vi "Check_Vol_Mounted.vi"(0 "Filename":path) -> (1 "Filename Out":path, 2 "exists?":bool)   [LabVIEW 2010]
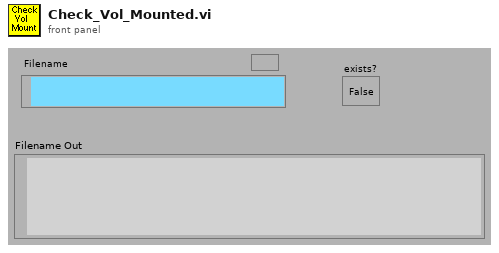
[diagram p1: front panel]
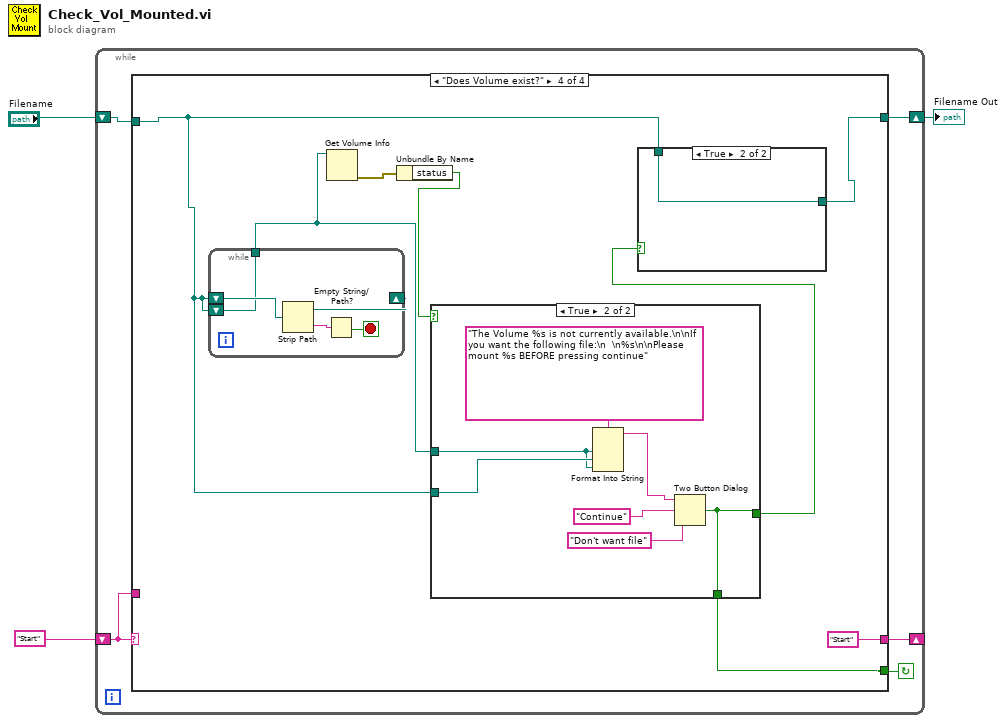
[diagram p0: block diagram]
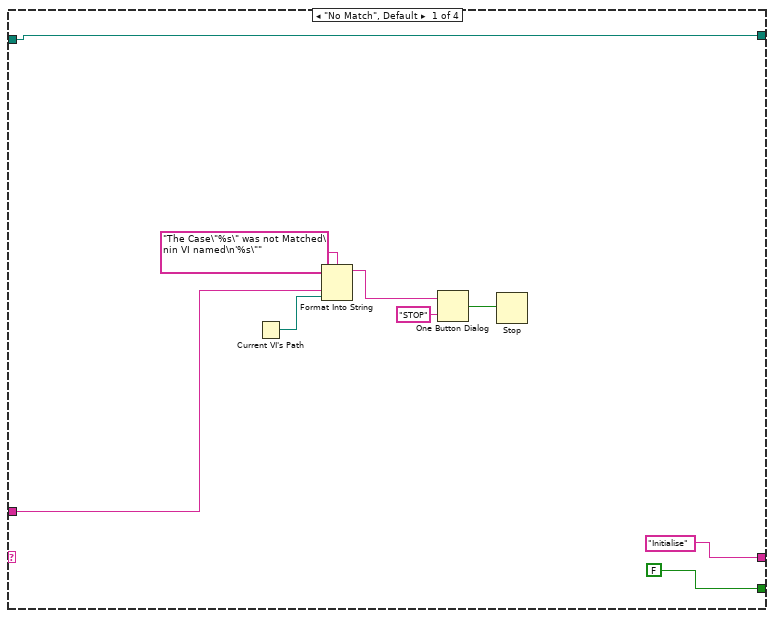
[diagram p2: hidden frame]
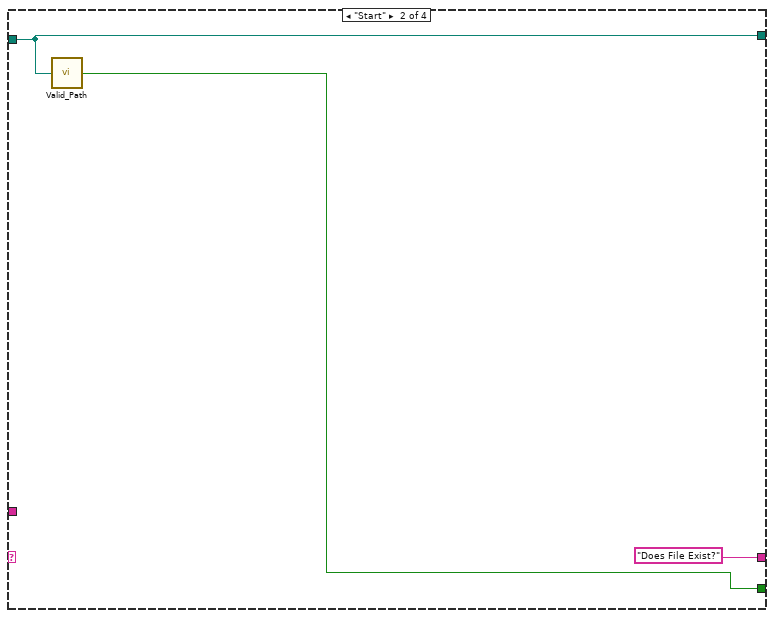
[diagram p3: hidden frame]
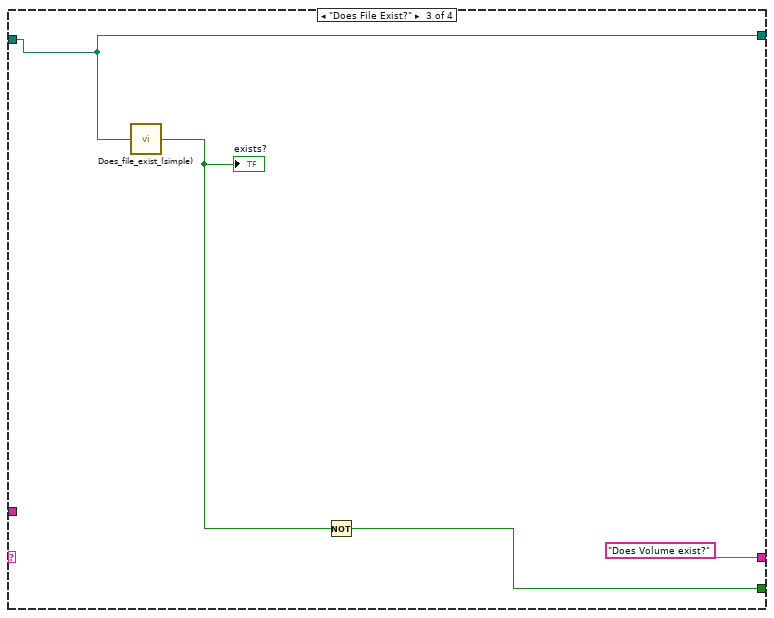
[diagram p4: hidden frame]
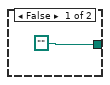
[diagram p5: hidden frame]
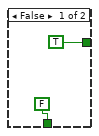
[diagram p6: hidden frame]
diagram:
  n1 = while {
    shift-left: "Start" -> [w6]
    shift-right: [w7] -> _
    shift-right: [w4] -> w1
    shift-left: "Filename" -> [w5]
    stop <- w8 continue-if-true
    n2 = case shown="\"Does Volume exist?\"" w6 {
      tunnel: [FALSE w19 w22 w26] -> w8
      tunnel: ["Initialise" "Does File Exist?" "Does Volume exist?" "Start"] -> w7
      tunnel: w6 -> [w12 _ _ _]
      tunnel: w5 -> [w9 w18 w21 w25]
      tunnel: [w9 w18 w21 w28] -> w4
      frame "No Match", Default {
        n3 = Current VI's Path() -> (path=w11:path)
        n4 = Format Into String(format string="The Case\"%s\" was not Matched\nin VI named\n'%s\"" ("Format String"), w12, w11) -> (resulting string=w15:string)  [unwired: 2 in, 1 out]
        n5 = One Button Dialog(message=w15, button name ("OK")="STOP") -> (true=w13:bool)
        n6 = Stop(stop? (T)=w13) -> ()
      }
      frame "Start" {
        n7 = call "Valid_Path.vi"("Filename"=w18) -> ("Valid Path?"=w19:bool)
      }
      frame "Does File Exist?" {
        n8 = call "Does_file_exist_(simple).vi"("Pathname"=w21) -> ("exists?"=w23:bool)
        "exists?" <- w23
        n9 = Not(x=w23) -> (.not. x?=w22:bool)
      }
      frame "Does Volume exist?" {
        n10 = while {
          shift-right: [w48] -> _
          shift-left: w25 -> [w46]
          shift-left: w25 -> [w45]
          tunnel: [w45] -> w29
          stop <- w44 stop-if-true
          n11 = Strip Path(path=w46) -> (stripped path=w48:path, name=w47:string)
          n12 = Empty String/Path?(string/path=w47) -> (empty?=w44:bool)
        }
        n13 = Get Volume Info(11:w29) -> (0:w31:errorcluster)  [unwired: 1 in, 5 out]
        n14 = Unbundle By Name(w31) -> ("status"=w30:bool)
        n15 = case shown="True" w30 {
          tunnel: w29 -> [_ w37]
          tunnel: [TRUE ("T button?") w39] -> w27
          tunnel: [FALSE ("T button?") w39] -> w26
          tunnel: w25 -> [_ w38]
          frame False {
          }
          frame True {
            n16 = Format Into String(format string="The Volume %s is not currently available.\n\nIf you want the following file:\n  \n%s\n\nPlease mount %s BEFORE pressing continue", w37, w38, w37) -> (resulting string=w42:string)  [unwired: 2 in, 1 out]
            n17 = Two Button Dialog(message=w42, 1:"Don't want file" ("F button name (\"Cancel\")"), 2:"Continue" ("T button name (\"OK\")")) -> (T button?=w39:bool)
          }
        }
        n18 = case shown="True" w27 {
          tunnel: [path "" w34] -> w28
          tunnel: w25 -> [_ w34]
          frame False {
          }
          frame True {
          }
        }
      }
    }
  }
  "Filename Out" <- w1
